vi "读取AGC.vi"(8 "error in (no error)":errorcluster) -> (0 "error out":errorcluster, 2 "(hi.lo)":u16)   [LabVIEW 2016]
panel:
  in  "vd_cmd_long_header_t":T1={"byCmdType"=20, "bySubCmd"=131, "byParam_h"=0, "byParam_l"=5, "byAddr1_hh"=0, "byAddr1_h"=0, "byAddr1_l"=0, "byAddr1_ll"=0, "byAddr2_hh"=0, "byAddr2_h"=0, "byAddr2_l"=0, "byAddr2_ll"=0, "byLen_hh"=0, "byLen_h"=0, "byLen_l"=0, "byLen_ll"=0}
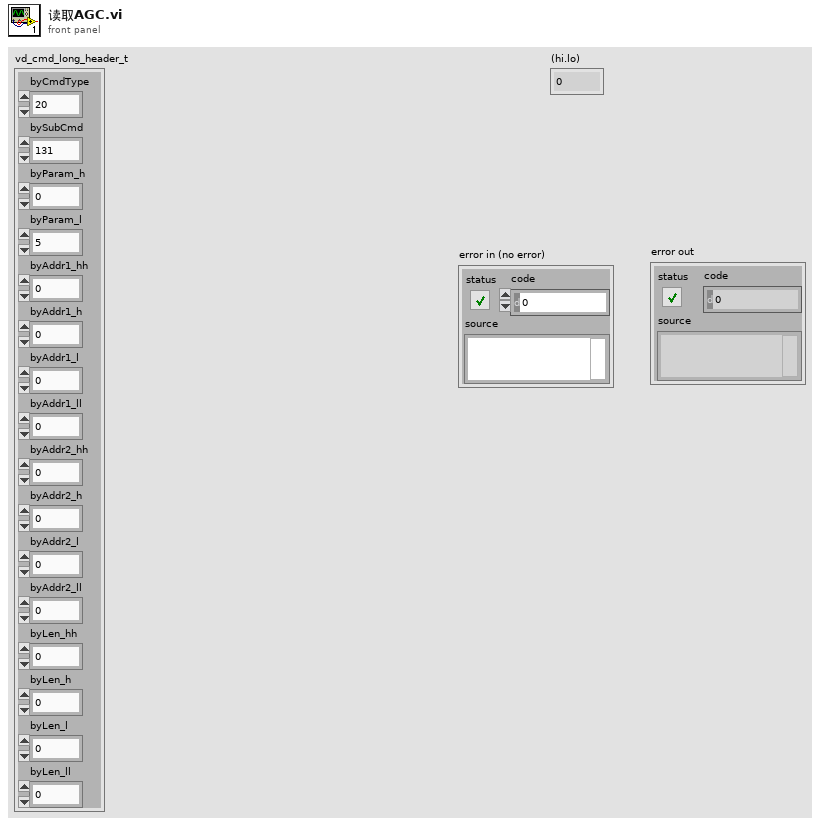
[diagram p1: front panel]
types:
  T1 = cluster{"byCmdType":u8, "bySubCmd":u8, "byParam_h":u8, "byParam_l":u8, "byAddr1_hh":u8, "byAddr1_h":u8, "byAddr1_l":u8, "byAddr1_ll":u8, "byAddr2_hh":u8, "byAddr2_h":u8, "byAddr2_l":u8, "byAddr2_ll":u8, "byLen_hh":u8, "byLen_h":u8, "byLen_l":u8, "byLen_ll":u8}
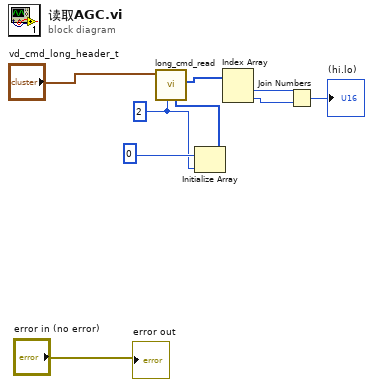
[diagram p0: block diagram]
diagram:
  w3 = u32 2 ("dwLen")
  n1 = Initialize Array(0, w3) -> (w2:i32[])
  n2 = call "long_cmd_read.vi"("data"=w2, "dwLen"=w3, "vd_cmd_long_header_t"="vd_cmd_long_header_t") -> ("data out"=w8:u8[])  [unwired: 6 in, 2 out]
  n3 = Index Array(array=w8) -> (element #1=w7:u8, element #2=w6:u8)  [unwired: 2 in]
  n4 = Join Numbers(hi=w7, lo=w6) -> ((hi.lo)=→"(hi.lo)":u16)
  "error out" <- "error in (no error)"
